vi "Gauge Block Classification.vi"(7 "블록삭제?(T)":bool=TRUE, 10 "블록리스트":string[](array[string]), 11 "게이지 블록 교정data":string[][](array[string])) -> (0 "불확도배열":string[](array[string]), 1 "열팽창계수":string, 2 "교정값(값)":dbl[](array[numeric]), 3 "블록치수":dbl[](array[numeric]), 4 "교정값(문자)":string[](array[string]), 6 "stop?":bool)   [LabVIEW 2020]
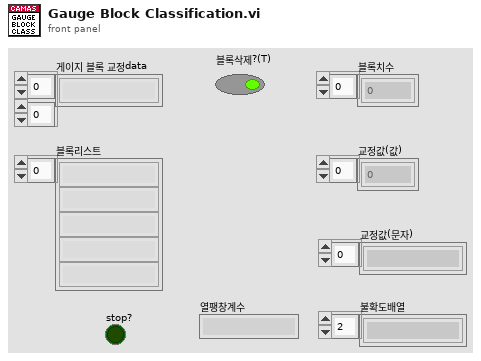
[diagram p1: front panel]
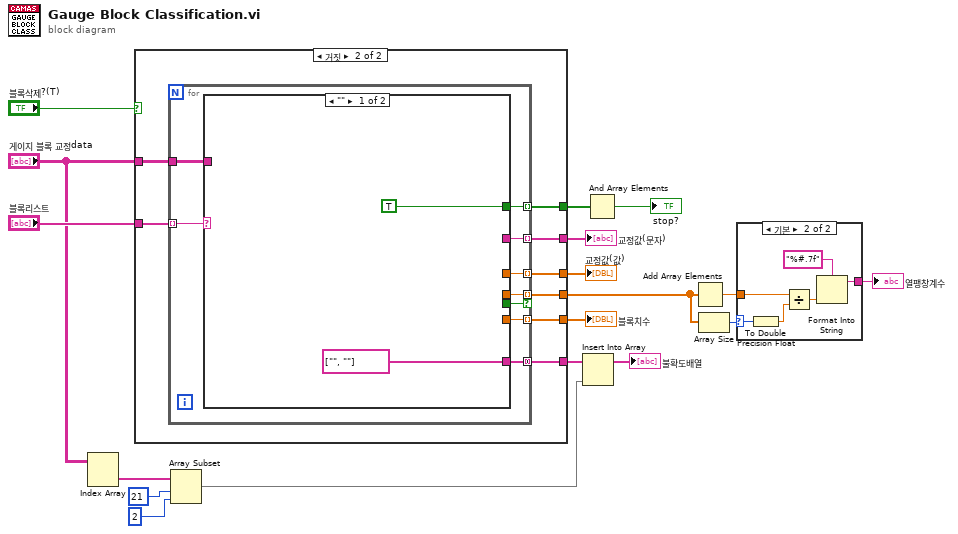
[diagram p0: block diagram]
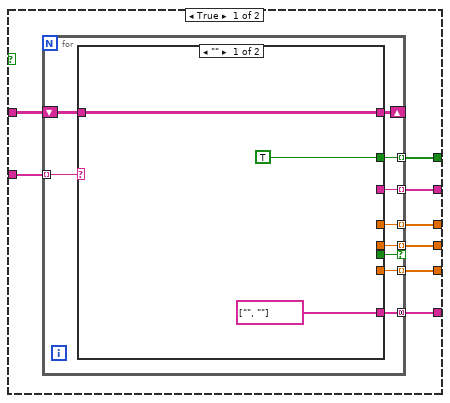
[diagram p2: hidden frame]
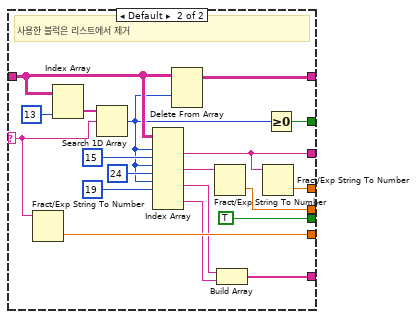
[diagram p3: hidden frame]
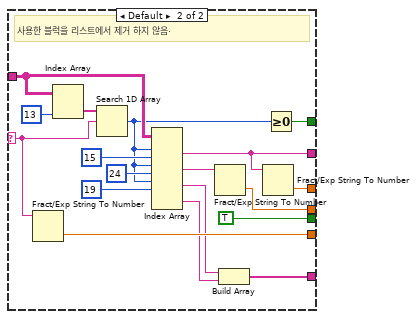
[diagram p4: hidden frame]
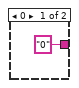
[diagram p5: hidden frame]
diagram:
  n1 = Index Array(array="게이지 블록 교정data") -> (element=w4:string[])  [unwired: 2 in]
  n2 = case shown="거짓" "블록삭제?(T)" {
    tunnel: [w26 w66] -> w18
    tunnel: [w25 w65] -> w17
    tunnel: "블록리스트" -> [w24 w64]
    tunnel: [w23 w63] -> w15
    tunnel: "게이지 블록 교정data" -> [w22 w60]
    tunnel: [w21 w62] -> w14
    tunnel: [w20 w61] -> w11
    tunnel: [w19 w59] -> w7
    frame True {
      n3 = for {
        tunnel: w24 -> [w35] mode=indexing
        tunnel: [w32] -> w21 mode=indexing
        tunnel: [w36] -> w23 mode=indexing
        shift-right: [w33] -> _
        shift-left: w22 -> [w34]
        tunnel: [w31] -> w25 mode=indexing
        tunnel: [w30] -> w26 mode=indexing
        tunnel: [w29] -> w20 mode=indexing if=w28
        tunnel: [w27] -> w19 mode=concatenating
        n4 = case shown="\"\"" w35 {
          selector: w35 -> [_ w52]
          tunnel: [TRUE w58] -> w32
          tunnel: [_ w50] -> w36
          tunnel: w34 -> [w38 w56]
          tunnel: [w38 w57] -> w33
          tunnel: [_ TRUE] -> w28
          tunnel: [_ w49] -> w31
          tunnel: [_ w48] -> w30
          tunnel: [_ w45] -> w29
          tunnel: [string[] ["", ""] w40] -> w27
          frame "" {
          }
          frame Default {
            # "사용한 블럭은 리스트에서 제거"
            n5 = Fract/Exp String To Number(string=w52) -> (number=w48:dbl)  [unwired: 3 in, 1 out]
            n6 = Index Array(array=w56, index (col)=13 ("비활성화된 인덱스 (열)")) -> (element=w55:string[])  [unwired: 1 in]
            n7 = Search 1D Array(1D array=w55, element=w52) -> (index of element=w44:i32)  [unwired: 1 in]
            n8 = Index Array(array=w56, index (row) #1=w44, index (col) #1=15 ("인덱스 (열)"), index (row) #2=w44, index (col) #2=24 ("인덱스 (열)"), index (row) #3=w44, index (col) #3=19 ("비활성화된 인덱스 (열)")) -> (element #1=w50:string, element #2=w46:string, element #3=w42:string, element #4=w41:string)  [unwired: 2 in]
            n9 = Delete From Array(array=w56, index (row)=w44) -> (array with subset deleted=w57:string[][])  [unwired: 2 in, 1 out]
            n10 = Fract/Exp String To Number(string=w46) -> (number=w45:dbl)  [unwired: 3 in, 1 out]
            n11 = Build Array(w42, w41) -> (w40:string[])
            n12 = Fract/Exp String To Number(string=w50) -> (number=w49:dbl)  [unwired: 3 in, 1 out]
            n13 = Greater Or Equal To 0?(x=w44) -> (x >= 0?=w58:bool)
          }
        }
      }
    }
    frame False {
      n14 = for {
        tunnel: w64 -> [w74] mode=indexing
        tunnel: [w73] -> w62 mode=indexing
        tunnel: [w75] -> w63 mode=indexing
        tunnel: [w72] -> w65 mode=indexing
        tunnel: [w71] -> w66 mode=indexing
        tunnel: [w70] -> w61 mode=indexing if=w69
        tunnel: w60 -> [w68]
        tunnel: [w67] -> w59 mode=concatenating
        n15 = case shown="\"\"" w74 {
          selector: w74 -> [_ w90]
          tunnel: [TRUE w95] -> w73
          tunnel: [_ w88] -> w75
          tunnel: w68 -> [_ w94]
          tunnel: [_ TRUE] -> w69
          tunnel: [_ w87] -> w72
          tunnel: [_ w86] -> w71
          tunnel: [_ w83] -> w70
          tunnel: [string[] ["", ""] w78] -> w67
          frame "" {
          }
          frame Default {
            # "사용한 블럭을 리스트에서 제거 하지 않음."
            n16 = Fract/Exp String To Number(string=w90) -> (number=w86:dbl)  [unwired: 3 in, 1 out]
            n17 = Index Array(array=w94, index (col)=13 ("비활성화된 인덱스 (열)")) -> (element=w93:string[])  [unwired: 1 in]
            n18 = Search 1D Array(1D array=w93, element=w90) -> (index of element=w82:i32)  [unwired: 1 in]
            n19 = Index Array(array=w94, index (row) #1=w82, index (col) #1=15 ("인덱스 (열)"), index (row) #2=w82, index (col) #2=24 ("인덱스 (열)"), index (row) #3=w82, index (col) #3=19 ("인덱스 (열)")) -> (element #1=w88:string, element #2=w84:string, element #3=w80:string, element #4=w79:string)  [unwired: 2 in]
            n20 = Fract/Exp String To Number(string=w84) -> (number=w83:dbl)  [unwired: 3 in, 1 out]
            n21 = Build Array(w80, w79) -> (w78:string[])
            n22 = Fract/Exp String To Number(string=w88) -> (number=w87:dbl)  [unwired: 3 in, 1 out]
            n23 = Greater Or Equal To 0?(x=w82) -> (x >= 0?=w95:bool)
          }
        }
      }
    }
  }
  "블록치수" <- w18
  "교정값(값)" <- w17
  "교정값(문자)" <- w15
  n24 = Array Subset(array=w4, index=21 ("길이"), length=2 ("인덱스")) -> (w3:string[])
  n25 = Insert Into Array(array=w7, new element=w3) -> (→"불확도배열":string[])  [unwired: 1 in]
  n26 = And Array Elements(Boolean array=w14) -> (logical AND=→"stop?":bool)
  n27 = Add Array Elements(numeric array=w11) -> (sum=w12:dbl)
  n28 = Array Size(array=w11) -> (size(s)=w9:i32)
  n29 = case shown="기본" w9 {
    selector: w9 -> [_ w97]
    tunnel: w12 -> [_ w102]
    tunnel: ["0" w98] -> w10
    frame 0 {
    }
    frame Default {
      n30 = To Double Precision Float(number=w97) -> (double precision float=w101:dbl)
      n31 = Divide(x=w102, y=w101) -> (x/y=w100:dbl)
      n32 = Format Into String(format string="%#.7f" ("포맷 문자열"), w100) -> (resulting string=w98:string)  [unwired: 2 in, 1 out]
    }
  }
  "열팽창계수" <- w10
